vi "ModeDrivebase.vi"(0 "Master State In":T1(ring)) -> (1 "Locked Heading (deg)":dbl=nan, 2 "Locked Y (in)":dbl=nan, 3 "Locked X (in)":dbl=nan)   [LabVIEW 2023]
doc: "This VI manages the robot drivebase mode. The default mode is driver control in which the swerve drive accepts all drive inputs and seemlessly combines them with autonomous assist controllers."
uses:
  <vilib>/Rock Robotics/WPI/DriverStation/WPI_DriverStationAllianceInfo.ctl
  05c444a4-6fa2-41d1-b82f-7624368f5fc5.vi
  294c1908-0ee9-4345-ab4e-8875c1d29428.vi
  989559c0-fd34-4975-afdb-c78bb7c8d441.vi
  c846a6c8-d51c-4150-87fb-7ec9fd787ba5.vi
  9e583775-f5ae-4d20-b542-91c1e1cefe2f.vi
  GlobalPoseAndTargeting.vi
  GlobalDrivebase.vi
  GlobalDriverStationCommands.vi
  GlobalShooter.vi
  GlobalDriverStationData.vi
panel:
  in  "Blue Stage Y":dbl=331.5 format="%#_13g"
  in  "Stage Y":dbl=28.5 format="%#_13g"
  in  "Truss center Y":dbl=158.0
  in  "Truss center X":dbl=192.0
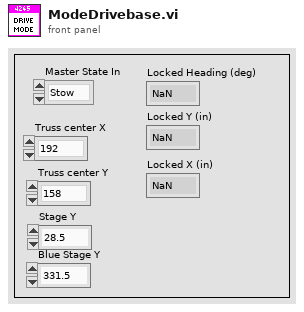
[diagram p1: front panel]
types:
  T1 = enum16{"Stow", "Speaker", "Amp", "Climbing", "Trap"}
  T2 = typedef "WPI_DriverStationAllianceInfo.ctl" = enum16{"Red", "Blue", "Invalid"}
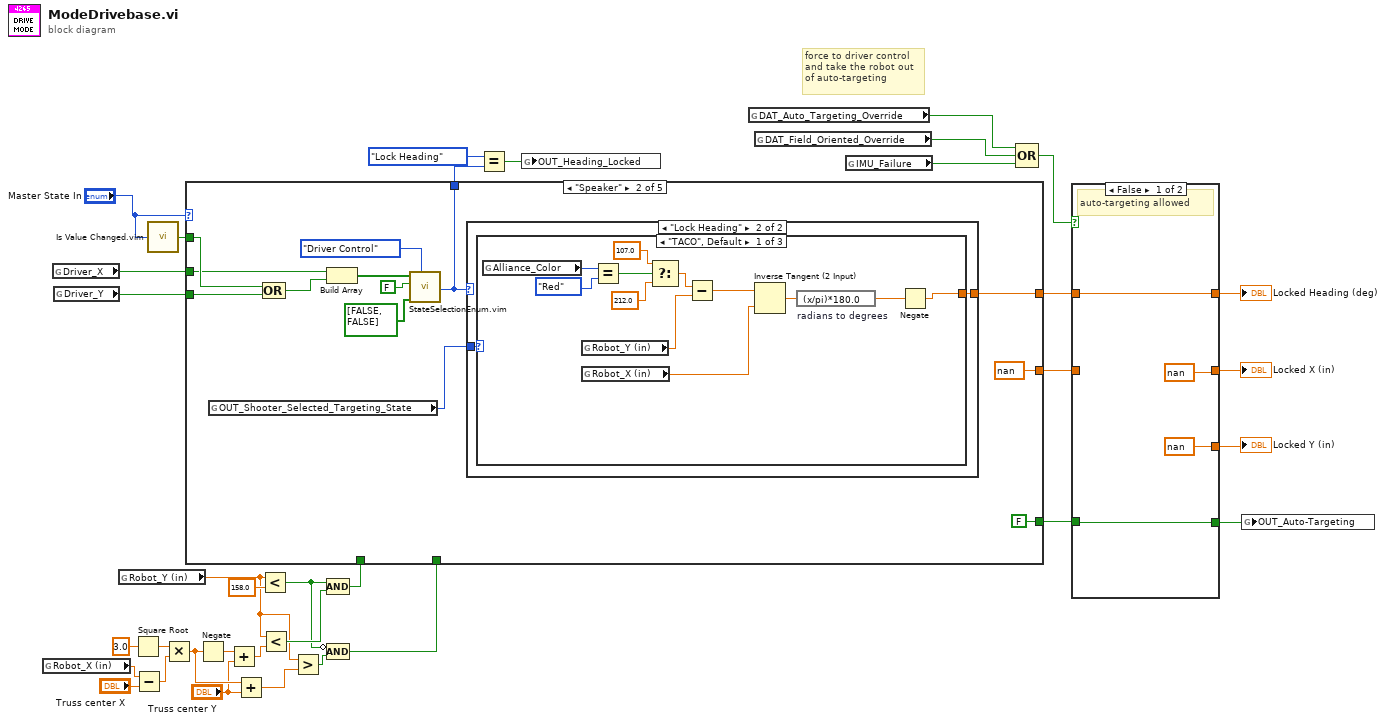
[diagram p0: block diagram]
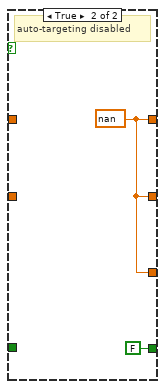
[diagram p2: hidden frame]
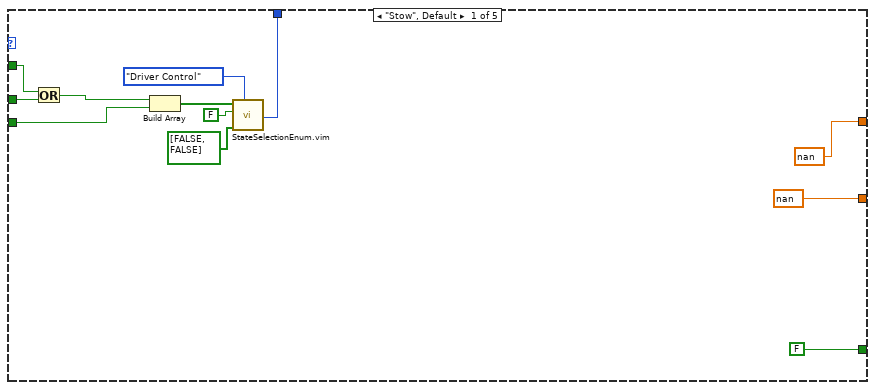
[diagram p3: hidden frame]
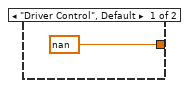
[diagram p4: hidden frame]
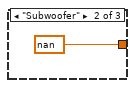
[diagram p5: hidden frame]
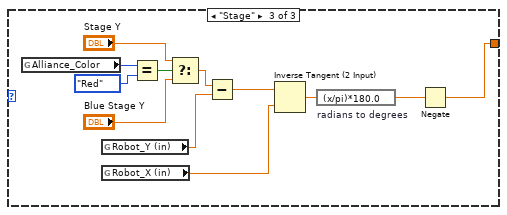
[diagram p6: hidden frame]
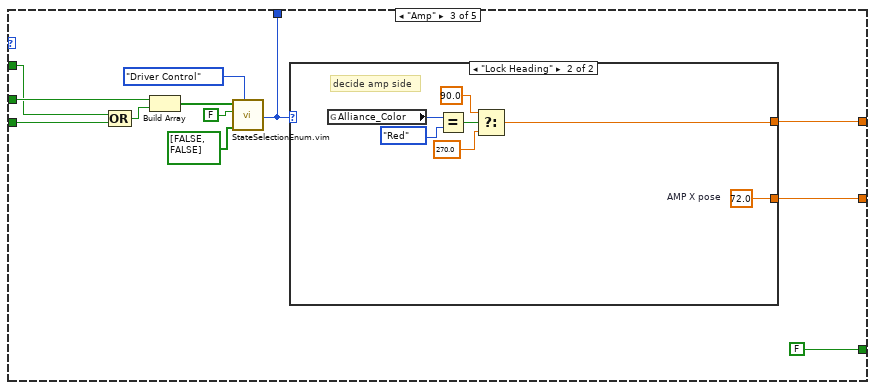
[diagram p7: hidden frame]
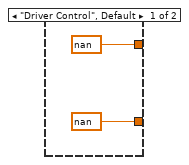
[diagram p8: hidden frame]
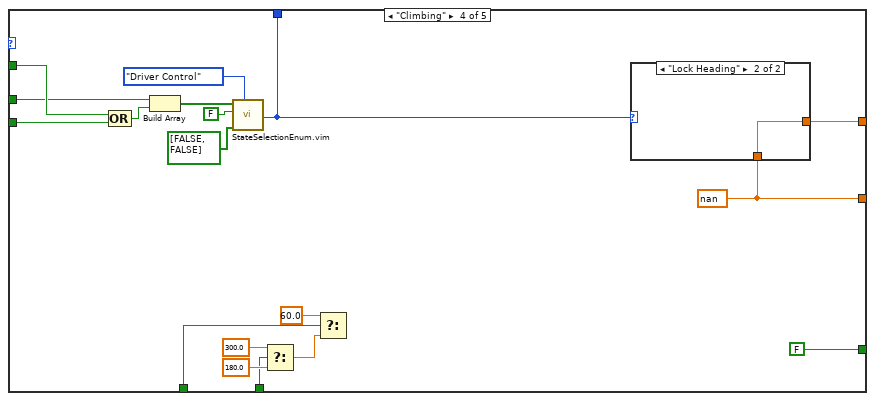
[diagram p9: hidden frame]
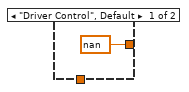
[diagram p10: hidden frame]
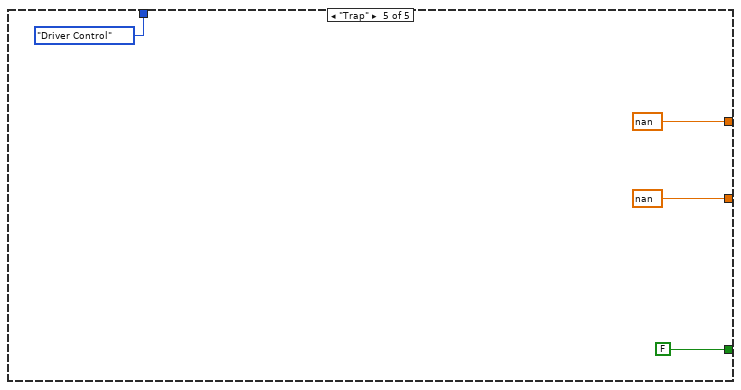
[diagram p11: hidden frame]
diagram:
  # "force to driver control\nand take the robot out\nof auto-targeting"
  n1 = global read "GlobalPoseAndTargeting.vi" "Robot_X (in)"() -> (w20:dbl)
  n2 = global read "GlobalDriverStationCommands.vi" "Driver_X"() -> (w26:bool)
  n3 = global read "GlobalDriverStationCommands.vi" "Driver_Y"() -> (w23:bool)
  n4 = global read "GlobalPoseAndTargeting.vi" "Robot_Y (in)"() -> (w9:dbl)
  n5 = Square Root(x=3.0) -> (sqrt(x)=w17:dbl)
  n6 = Subtract(x=w20, y="Truss center X") -> (x-y=w18:dbl)
  n7 = call "Is Value Changed.vim"("value"="Master State In") -> ("changed or first call?"=w24:bool)
  n8 = Multiply(x=w17, y=w18) -> (x*y=w12:dbl)
  n9 = Negate(x=w12) -> (-x=w16:dbl)
  n10 = Add(x=w16, y="Truss center Y") -> (x+y=w15:dbl)
  n11 = Add(x=w12, y="Truss center Y") -> (x+y=w10:dbl)
  n12 = Less?(x=w9, y=158.0) -> (x < y?=w13:bool)
  n13 = Less?(x=w9, y=w15) -> (x < y?=w14:bool)
  n14 = Greater?(x=w9, y=w10) -> (0:w8:bool)
  n15 = Compound Arithmetic op=AND(w13, w14) -> (w7:bool)
  n16 = Compound Arithmetic op=AND(invert w13, w8) -> (w6:bool)
  n17 = case shown="\"Speaker\"" "Master State In" {
    tunnel: [nan w51 w89 w112 nan] -> w31
    tunnel: [FALSE FALSE FALSE FALSE FALSE] -> w28
    tunnel: w26 -> [w42 w54 w95 w114 _]
    tunnel: w24 -> [w43 w55 w94 w115 _]
    tunnel: w23 -> [w38 w53 w93 w113 _]
    tunnel: w7 -> [_ _ _ w117 _]
    tunnel: w6 -> [_ _ _ w116 _]
    tunnel: [w40 w50 w91 w111 enum16{"Driver Control", "Lock Heading"}."Driver Control" ("Selected State")] -> w5
    tunnel: [nan nan w90 w110 nan] -> w2
    frame "Stow", Default {
      n18 = Or(x=w43, y=w42) -> (x .or. y?=w41:bool)
      n19 = Build Array(w41, w38) -> (w47:bool[])
      n20 = call "StateSelectionEnum.vim"("Enum Def"=enum16{"Driver Control", "Lock Heading"}."Driver Control" ("Drive Mode"), "Disallowed States"=bool[] [FALSE, FALSE], "Enable Edge Trigger"=FALSE, "State Triggers"=w47) -> ("Selected State"=w40:enum16{"Driver Control", "Lock Heading"})  [unwired: 1 in, 1 out]
    }
    frame "Speaker" {
      n21 = global read "GlobalShooter.vi" "OUT_Shooter_Selected_Targeting_State"() -> (w48:enum16{"TACO", "Subwoofer", "Stage"})
      n22 = Compound Arithmetic op=OR(w55, w53) -> (w60:bool)
      n23 = Build Array(w54, w60) -> (w59:bool[])
      n24 = call "StateSelectionEnum.vim"("Enum Def"=enum16{"Driver Control", "Lock Heading"}."Driver Control" ("Drive Mode"), "Disallowed States"=bool[] [FALSE, FALSE], "Enable Edge Trigger"=FALSE, "State Triggers"=w59) -> ("Selected State"=w50:enum16{"Driver Control", "Lock Heading"})  [unwired: 1 in, 1 out]
      n25 = case shown="\"Lock Heading\"" w50 {
        tunnel: [nan w63] -> w51
        tunnel: w48 -> [_ w62]
        frame "Driver Control", Default {
        }
        frame "Lock Heading" {
          n26 = case shown="\"TACO\", Default" w62 {
            tunnel: [w64 nan w77] -> w63
            frame "TACO", Default {
              n27 = global read "GlobalDriverStationData.vi" "Alliance_Color"() -> (w74:T2)
              n28 = global read "GlobalPoseAndTargeting.vi" "Robot_Y (in)"() -> (w68:dbl)
              n29 = global read "GlobalPoseAndTargeting.vi" "Robot_X (in)"() -> (w67:dbl)
              n30 = Equal?(x=w74, y=WPI_DriverStationAllianceInfo."Red") -> (x = y?=w71:bool)
              n31 = Select(t=107.0 ("Robot_Y (in)"), s=w71, f=212.0 ("Robot_Y (in)")) -> (s? t:f=w69:dbl)
              n32 = Subtract(x=w69, y=w68) -> (x-y=w66:dbl)
              n33 = Inverse Tangent (2 Input)(1:w67, 2:w66) -> (0:w70:dbl)
              n34 = expression code="(x/pi)*180.0" "radians to degrees"(w70) -> (w65:dbl)
              n35 = Negate(x=w65) -> (-x=w64:dbl)
            }
            frame "Subwoofer" {
            }
            frame "Stage" {
              n36 = global read "GlobalDriverStationData.vi" "Alliance_Color"() -> (w88:T2)
              n37 = global read "GlobalPoseAndTargeting.vi" "Robot_Y (in)"() -> (w82:dbl)
              n38 = global read "GlobalPoseAndTargeting.vi" "Robot_X (in)"() -> (w81:dbl)
              n39 = Equal?(x=w88, y=WPI_DriverStationAllianceInfo."Red") -> (x = y?=w86:bool)
              n40 = Select(t="Stage Y", s=w86, f="Blue Stage Y") -> (s? t:f=w78:dbl)
              n41 = Subtract(x=w78, y=w82) -> (x-y=w80:dbl)
              n42 = Inverse Tangent (2 Input)(1:w81, 2:w80) -> (0:w83:dbl)
              n43 = expression code="(x/pi)*180.0" "radians to degrees"(w83) -> (w79:dbl)
              n44 = Negate(x=w79) -> (-x=w77:dbl)
            }
          }
        }
      }
    }
    frame "Amp" {
      n45 = Compound Arithmetic op=OR(w94, w93) -> (w92:bool)
      n46 = Build Array(w95, w92) -> (w99:bool[])
      n47 = call "StateSelectionEnum.vim"("Enum Def"=enum16{"Driver Control", "Lock Heading"}."Driver Control" ("Drive Mode"), "Disallowed States"=bool[] [FALSE, FALSE], "Enable Edge Trigger"=FALSE, "State Triggers"=w99) -> ("Selected State"=w91:enum16{"Driver Control", "Lock Heading"})  [unwired: 1 in, 1 out]
      n48 = case shown="\"Lock Heading\"" w91 {
        tunnel: [nan w103] -> w89
        tunnel: [nan w104] -> w90
        frame "Driver Control", Default {
        }
        frame "Lock Heading" {
          w104 = 72.0  # AMP X pose
          # "decide amp side"
          n49 = global read "GlobalDriverStationData.vi" "Alliance_Color"() -> (w105:T2)
          n50 = Equal?(x=w105, y=WPI_DriverStationAllianceInfo."Red") -> (x = y?=w108:bool)
          n51 = Select(t=90.0, s=w108, f=270.0) -> (s? t:f=w103:dbl)
        }
      }
    }
    frame "Climbing" {
      w110 = nan
      n52 = Compound Arithmetic op=OR(w115, w113) -> (w123:bool)
      n53 = Build Array(w114, w123) -> (w127:bool[])
      n54 = call "StateSelectionEnum.vim"("Enum Def"=enum16{"Driver Control", "Lock Heading"}."Driver Control" ("Drive Mode"), "Disallowed States"=bool[] [FALSE, FALSE], "Enable Edge Trigger"=FALSE, "State Triggers"=w127) -> ("Selected State"=w111:enum16{"Driver Control", "Lock Heading"})  [unwired: 1 in, 1 out]
      n55 = Select(t=300.0, s=w116, f=180.0) -> (s? t:f=w122:dbl)
      n56 = Select(t=60.0, s=w117, f=w122) -> ()  [unwired: 1 out]
      n57 = case shown="\"Lock Heading\"" w111 {
        tunnel: [nan w129] -> w112
        tunnel: w110 -> [_ w129]
        frame "Driver Control", Default {
        }
        frame "Lock Heading" {
        }
      }
    }
    frame "Trap" {
    }
  }
  n58 = Equal?(x=enum16{"Driver Control", "Lock Heading"}."Lock Heading", y=w5) -> (x = y?=w3:bool)
  n59 = global write "GlobalDrivebase.vi" "OUT_Heading_Locked"(w3) -> ()
  n60 = global read "GlobalDrivebase.vi" "DAT_Auto_Targeting_Override"() -> (w33:bool)
  n61 = global read "GlobalDrivebase.vi" "DAT_Field_Oriented_Override"() -> (w34:bool)
  n62 = global read "GlobalPoseAndTargeting.vi" "IMU_Failure"() -> (w35:bool)
  n63 = Compound Arithmetic op=OR(w33, w34, w35) -> (w32:bool)
  n64 = case shown="False" w32 {
    tunnel: w31 -> [w135 _]
    tunnel: [w135 w139] -> w30
    tunnel: [nan w139] -> w1
    tunnel: [nan w139] -> w27
    tunnel: [w137 FALSE] -> w29
    tunnel: w28 -> [w137 _]
    tunnel: w2 -> [_ _]
    frame False {
      # "auto-targeting allowed"
    }
    frame True {
      w139 = nan
      # "auto-targeting disabled"
    }
  }
  "Locked Heading (deg)" <- w30
  "Locked Y (in)" <- w27
  "Locked X (in)" <- w1
  n65 = global write "GlobalDrivebase.vi" "OUT_Auto-Targeting"(w29) -> ()
